vi "training_rating_display_sub_v3.vi"(10 "Boolean":bool, 11 "Numeric":i32) -> ()   [LabVIEW 2020]
panel:
  out "String 2":string caption="String"
  out "Cluster 5":T1
  out "Cluster 4":T1
  out "String":string
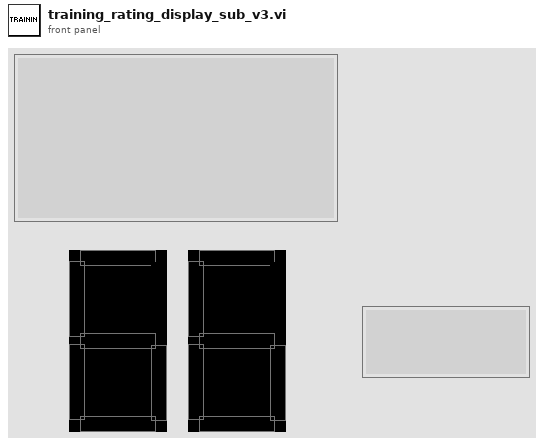
[diagram p1: front panel]
types:
  T1 = cluster{"Boolean":bool, "Boolean 2":bool, "Boolean 3":bool, "Boolean 4":bool, "Boolean 5":bool, "Boolean 6":bool, "Boolean 7":bool}
  T2 = cluster{"t[0]":bool, "t[1]":bool, "t[2]":bool, "t[3]":bool, "t[4]":bool, "t[5]":bool, "t[6]":bool}
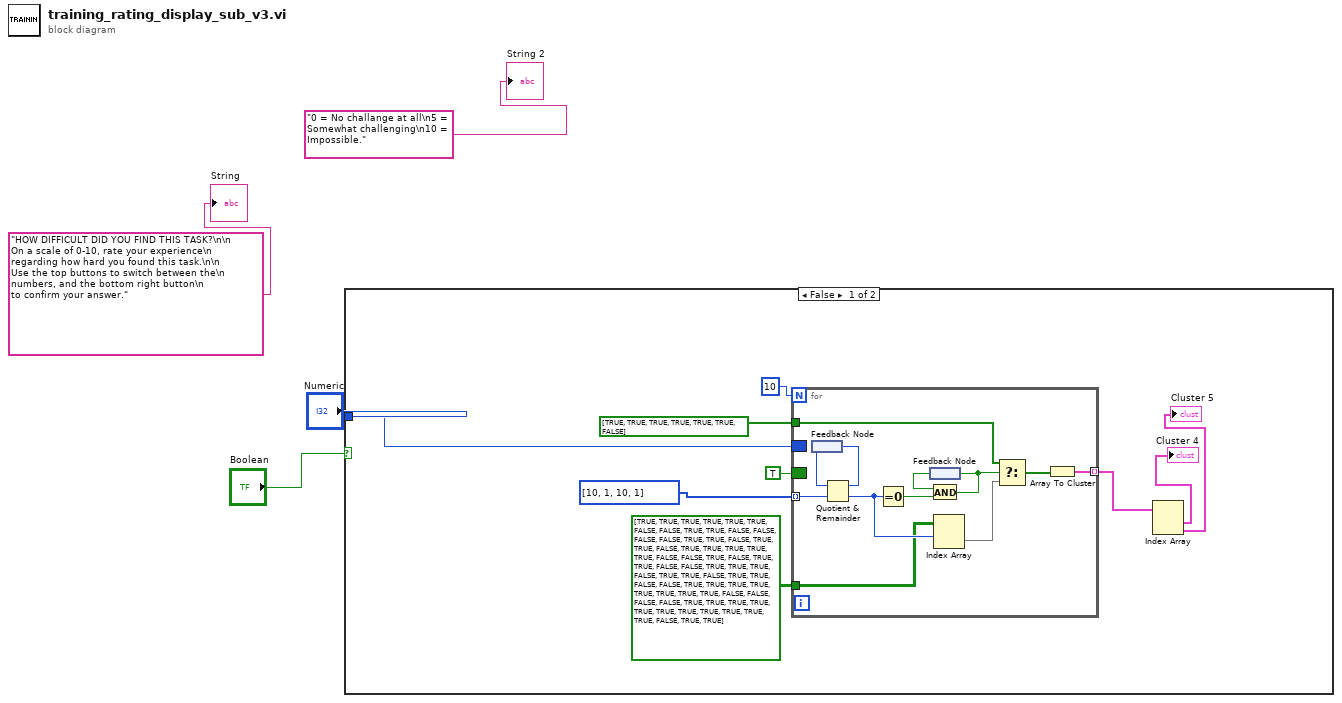
[diagram p0: block diagram]
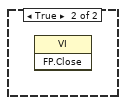
[diagram p2: hidden frame]
diagram:
  n1 = case shown="False" "Boolean" {
    tunnel: "Numeric" -> [w5 _]
    frame False {
      n2 = for {
        N: 10 -> [_]
        border: w5 -> [_]
        tunnel: i32[] [10, 1, 10, 1] -> [w23] mode=indexing
        tunnel: [w22] -> w8 mode=indexing
        border: TRUE -> [_]
        tunnel: bool[][] [[TRUE, TRUE, TRUE, TRUE, TRUE, TRUE, FALSE], [FALSE, TRUE, TRUE, FALSE, FALSE, FALSE, FALSE], [TRUE, TRUE, FALSE, TRUE, TRUE, FALSE, TRUE], [TRUE, TRUE, TRUE, TRUE, FALSE, FALSE, TRUE], [FALSE, TRUE, TRUE, FALSE, FALSE, TRUE, TRUE], [TRUE, FALSE, TRUE, TRUE, FALSE, TRUE, TRUE], [FALSE, FALSE, TRUE, TRUE, TRUE, TRUE, TRUE], [TRUE, TRUE, TRUE, FALSE, FALSE, FALSE, FALSE], [TRUE, TRUE, TRUE, TRUE, TRUE, TRUE, TRUE], [TRUE, TRUE, TRUE, TRUE, FALSE, TRUE, TRUE]] -> [w15]
        tunnel: bool[] [TRUE, TRUE, TRUE, TRUE, TRUE, TRUE, FALSE] ("t") -> [w14]
        n3 = feedback #1() -> (w24:i32)
        n4 = Quotient & Remainder(x=w24, y=w23) -> (x-y*floor(x/y)=w25:i32, floor(x/y)=w21:i32)
        n5 = feedback-in #1(w25) -> ()
        n6 = Equal To 0?(x=w21) -> (x = 0?=w20:bool)
        n7 = feedback #2() -> (w19:bool)
        n8 = And(x=w19, y=w20) -> (x .and. y?=w16:bool)
        n9 = feedback-in #2(w16) -> ()
        n10 = Index Array(array=w15, index (row)=w21) -> (element=w18:bool[])  [unwired: 1 in]
        n11 = Select(t=w14, s=w16, f=w18) -> (s? t:f=w17:bool[])
        n12 = Array To Cluster(array=w17) -> (cluster=w22:T2)
      }
      n13 = Index Array(array=w8) -> (element #1=→"Cluster 4":T2, element #2=→"Cluster 5":T2)  [unwired: 2 in]
    }
    frame True {
      n14 = invoke class="VI" method="FP.Close"() -> ()  [unwired: 3 in, 3 out]
    }
  }
  "String" <- "HOW DIFFICULT DID YOU FIND THIS TASK?\n\n       On a scale of 0-10, rate your experience\n        regarding how hard you found this task.\n\n        Use the top buttons to switch between the\n          numbers, and the bottom right button\n                   to confirm your answer."
  "String 2" <- "0 = No challange at all\n5 = Somewhat challenging\n10 = Impossible."
